vi "ep_Internal Parameters for Speed Estimation.vi"() -> (3 "internal parameters for speed estimation":T1)   [LabVIEW 2014, in "NI_EP_Motor Monitoring.lvlib"]
uses:
  <vilib>/addons/Electrical Power/Motor Monitoring/NI_EP_Motor Monitoring.lvlib
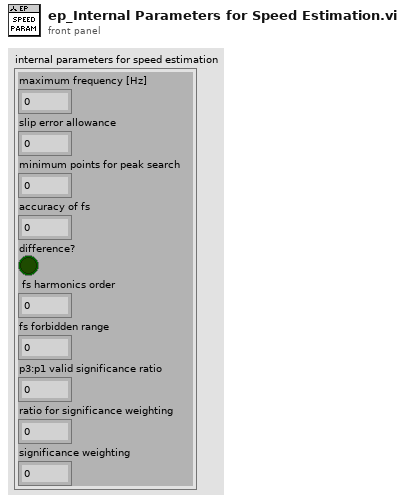
[diagram p1: front panel]
types:
  T1 = cluster{"maximum frequency [Hz]":dbl, "slip error allowance":dbl, "minimum points for peak search":dbl, "accuracy of fs":dbl, "difference?":bool, " fs harmonics order":i32, "fs forbidden range":dbl, "p3:p1 valid significance ratio":dbl, "ratio for significance weighting":dbl, "significance weighting":dbl}
  T2 = cluster{"maximum frequency [Hz]":dbl, "nameplate slip error allowance":dbl, "minimum points for peak search":dbl, "accuracy of fs":dbl, "difference?":bool, " fs harmonics order":i32, "fs forbidden range [Hz]":dbl, "p3:p1 valid significance ratio":dbl, "ratio for significance weighting":dbl, "significance weighting":dbl}
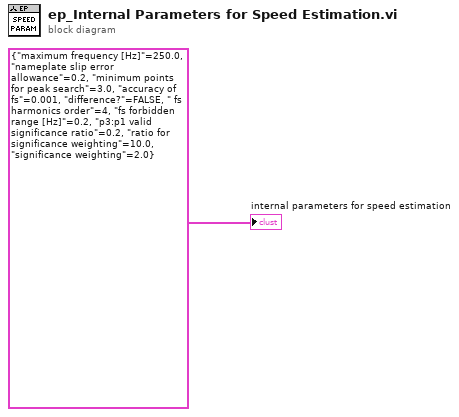
[diagram p0: block diagram]
diagram:
  "internal parameters for speed estimation" <- T2 {"maximum frequency [Hz]"=250.0, "nameplate slip error allowance"=0.2, "minimum points for peak search"=3.0, "accuracy of fs"=0.001, "difference?"=FALSE, " fs harmonics order"=4, "fs forbidden range [Hz]"=0.2, "p3:p1 valid significance ratio"=0.2, "ratio for significance weighting"=10.0, "significance weighting"=2.0} ("internal parameters for speed estimation")
